vi "LSX Get BPZ Joyspeed.vi"(8 "error in (no error)":errorcluster, 9 "pdAValue":dbl, 10 "lAPar":i32, 11 "lLSID":i32) -> (0 "error out":errorcluster, 1 "pdAValue out":dbl, 3 "function return":i32)   [LabVIEW 2018, in "Tango.lvlib"]
doc: "TANGOAPI int TANGOCALL LSX_GetBPZJoyspeed (int lLSID, int lAPar, double *pdAValue);"
uses:
  <userlib>/Tango/Tango.lvlib
  <userlib>/Tango/Tango_DLL.dll
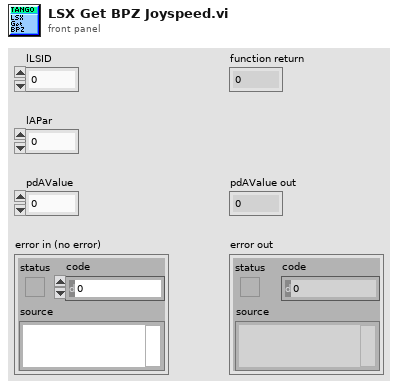
[diagram p1: front panel]
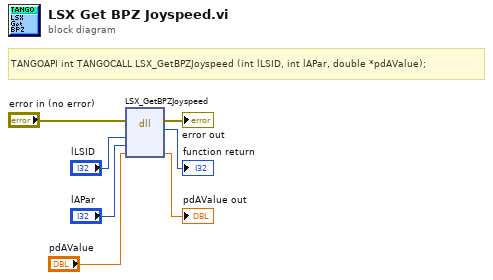
[diagram p0: block diagram]
diagram:
  # "TANGOAPI int TANGOCALL LSX_GetBPZJoyspeed (int lLSID, int lAPar, double *pdAValue);"
  n1 = dll-call lib="C:/Program Files (x86)/National Instruments/LabVIEW 2018/user.lib/Tango/Tango_DLL.*" fn="LSX_GetBPZJoyspeed"(error in="error in (no error)", "lLSID"="lLSID", "lAPar"="lAPar", "pdAValue"="pdAValue") -> (error out=→"error out":errorcluster, →"function return":i32, "pdAValue"=→"pdAValue out":dbl)  [unwired: 4 in, 1 out]
